vi "PMBus Read Byte Ext.vi"(0 "DevType":i32, 1 "CommandCodeExt":u8, 2 "PEC":u8, 5 "DevIndex":i32, 7 "PMBusIndex":i32, 9 "SlaveAddr":u8, 11 "error in (no error)":errorcluster, 12 "CommandCode":u8) -> (4 "pData":string, 6 "function return":i32, 15 "error out":errorcluster)   [LabVIEW 2012, in "ControlPMBus.lvlib"]
doc: "int WINAPI PMBus_ReadByteExt(int DevType,int DevIndex,int PMBusIndex,unsigned char SlaveAddr,unsigned char CommandCodeExt,unsigned char CommandCode, unsigned char *pData,unsigned char PEC);"
uses:
  ControlPMBus.lvlib
  Ginkgo_Driver.dll
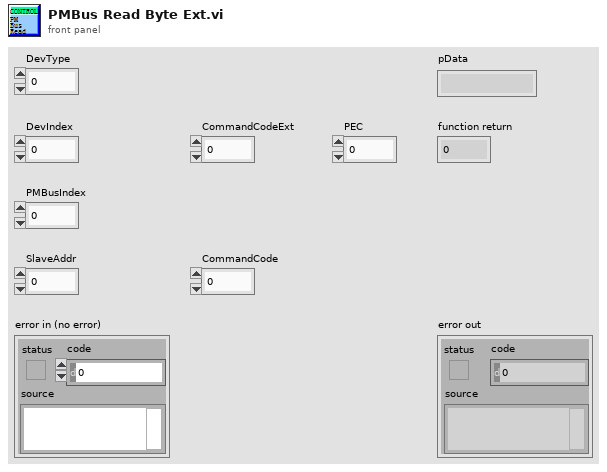
[diagram p1: front panel]
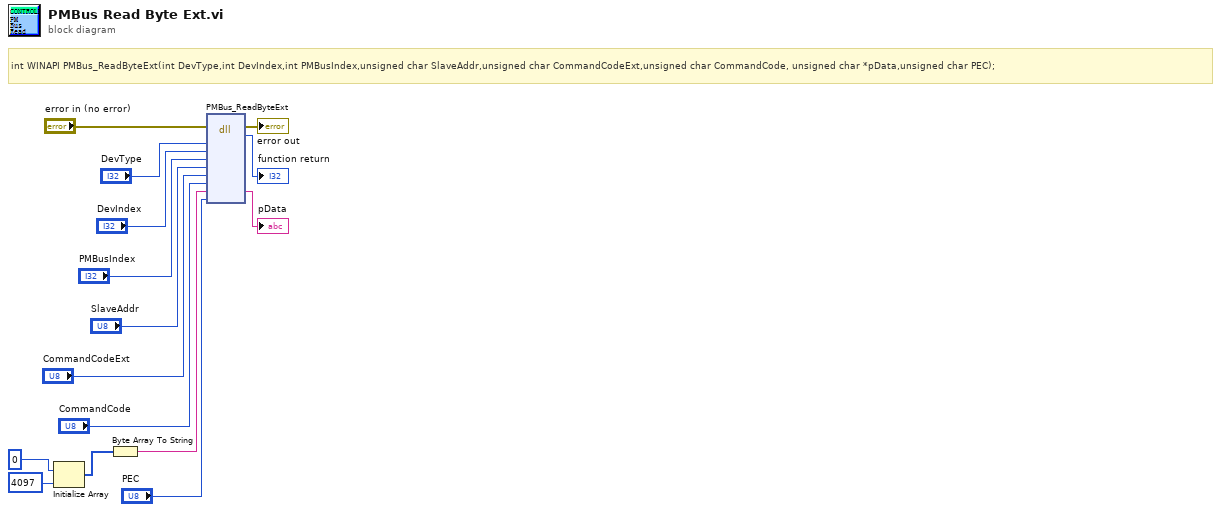
[diagram p0: block diagram]
diagram:
  # "int WINAPI PMBus_ReadByteExt(int DevType,int DevIndex,int PMBusIndex,unsigned char SlaveAddr,unsigned char CommandCodeExt,unsigned char CommandCode, unsigned char *pData,unsigned char PEC);"
  n1 = Initialize Array(u8 0 ("element"), 4097 ("dimension size")) -> (w8:u8[])
  n2 = Byte Array To String(unsigned byte array=w8) -> (string=w7:string)
  n3 = dll-call lib="E:/Project/vt_ginkgo/truck/Ginkgo Driver/vs2010/Ginkgo_USB-I2C_API_v2.0.3.0/lib/labview_32bit/ControlPMBus/Ginkgo_Driver.*" fn="PMBus_ReadByteExt"(error in="error in (no error)", "DevType"="DevType", "DevIndex"="DevIndex", "PMBusIndex"="PMBusIndex", "SlaveAddr"="SlaveAddr", "CommandCodeExt"="CommandCodeExt", "CommandCode"="CommandCode", "pData"=w7, "PEC"="PEC") -> (error out=→"error out":errorcluster, →"function return":i32, "pData"=→"pData":string)  [unwired: 9 in, 1 out]
